vi "Configure Event Callbacks.vi"(8 "error in (no error)":errorcluster, 10 "User Parameters":T1, 11 "Application Manager":refnum<k7>) -> (0 "error out":errorcluster, 3 "Event Callback Refnum Out":refnum<k27>)   [LabVIEW 2010, in "TS Simple LabVIEW OI Dependencies.lvlib"]
uses:
  TS Simple LabVIEW OI Dependencies.lvlib
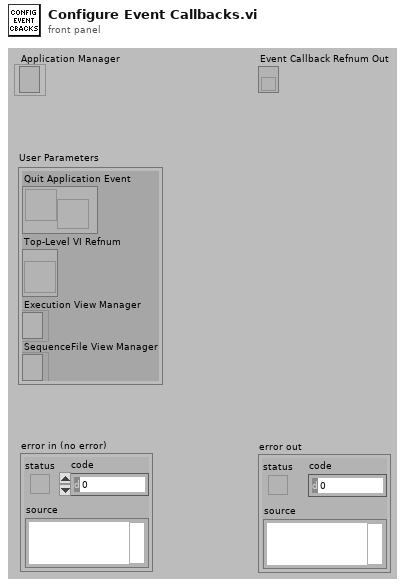
[diagram p1: front panel]
types:
  T1 = cluster{"Quit Application Event":refnum<user-event>, "Top-Level VI Refnum":refnum<vi>, "Execution View Manager":refnum<k7>, "SequenceFile View Manager":refnum<k7>}
  T2 = cluster{"Execution View Manager":refnum<k7>, "Top-Level VI Refnum":refnum<vi>}
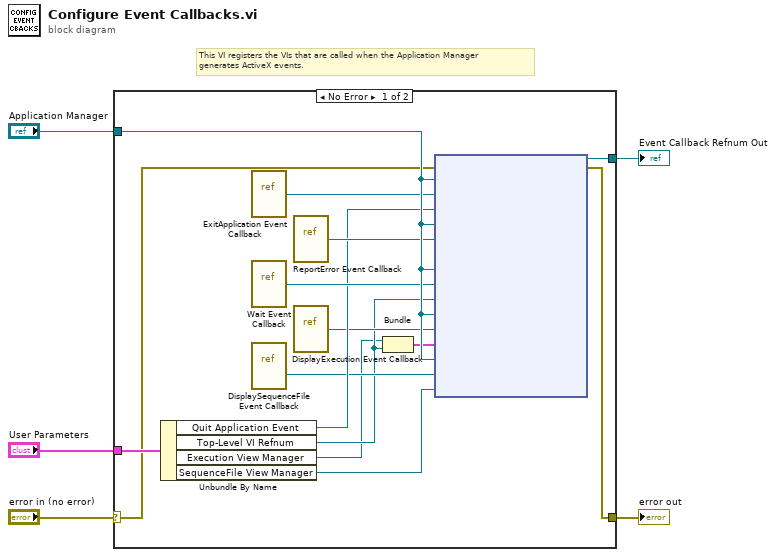
[diagram p0: block diagram]
diagram:
  # "This VI registers the VIs that are called when the Application Manager\ngenerates ActiveX events."
  n1 = case shown="No Error" "error in (no error)" {
    selector: "error in (no error)" -> [w12 w21]
    tunnel: "Application Manager" -> [w20 _]
    tunnel: [w19 _] -> w4
    tunnel: "User Parameters" -> [w15 _]
    tunnel: [w11 w21] -> w1
    frame No Error {
      n2 = Unbundle By Name(w15) -> ("Quit Application Event"=w14:refnum<user-event>, "Top-Level VI Refnum"=w7:refnum<vi>, "Execution View Manager"=w6:refnum<k7>, "SequenceFile View Manager"=w13:refnum<k7>)
      n3 = vi-ref "ExitApplication Event Callback.vi"() -> ("vi reference"=w16:refnum<vi>)
      n4 = vi-ref "Wait Event Callback.vi"() -> ("vi reference"=w18:refnum<vi>)
      n5 = vi-ref "DisplaySequenceFile Event Callback.vi"() -> ("vi reference"=w9:refnum<vi>)
      n6 = vi-ref "ReportError Event Callback.vi"() -> ("vi reference"=w17:refnum<vi>)
      n7 = vi-ref "DisplayExecution Event Callback.vi"() -> ("vi reference"=w10:refnum<vi>)
      n8 = Bundle("Execution View Manager"=w6, "Top-Level VI Refnum"=w7) -> (w8:T2)  [unwired: 1 out]
      n9 = node(w12, w20, w16, w14, w20, w17, w20, w18, w7, w20, w10, w8, w20, w9, w13) -> (w19:refnum<k27>, w11:errorcluster)  [unwired: 2 in]
    }
    frame Error {
    }
  }
  "Event Callback Refnum Out" <- w4
  "error out" <- w1
